vi "Read Cal Data.vi"(5 "NewOffsets(V)":dbl[](array[numeric]), 11 "error in (no error)":errorcluster, 12 "Enum":enum16{"Init", "Read", "Write"}(ring)) -> (4 "AllowZero":bool[](array[boolean]), 6 "Slope":dbl[](array[numeric]), 8 "Offset":dbl[](array[numeric]), 10 "Channel Names":string[](array[string]), 15 "error out":errorcluster)   [LabVIEW 2018]
uses:
  <vilib>/Utility/file.llb/Read Delimited Spreadsheet (string).vi
  <vilib>/Utility/file.llb/Write Delimited Spreadsheet (string).vi
panel:
  out "all rows":string[][](array[string])
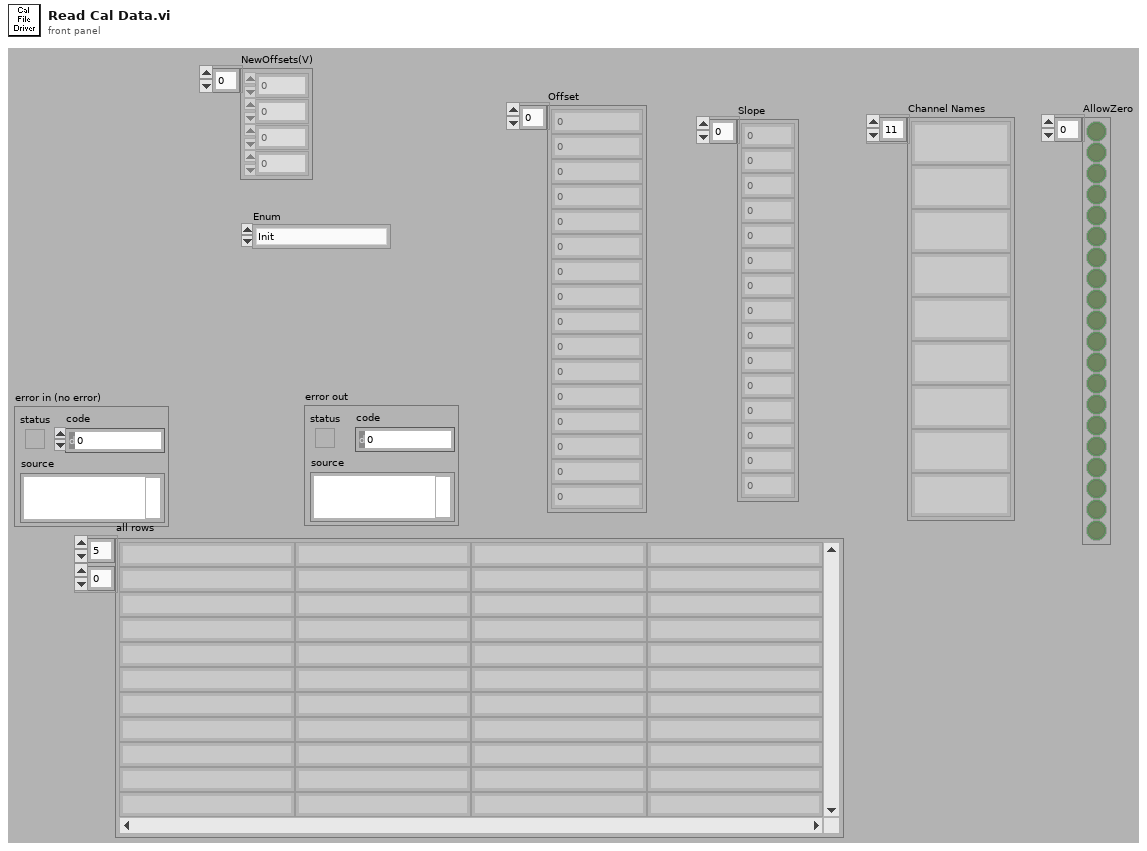
[diagram p1: front panel]
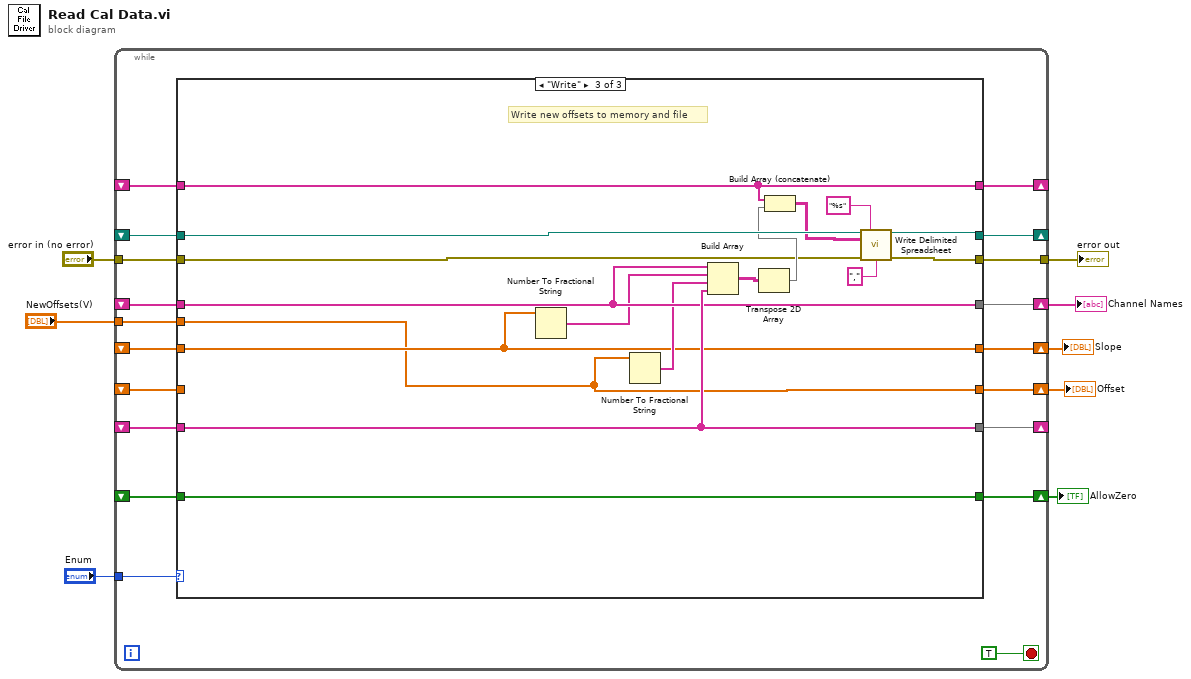
[diagram p0: block diagram]
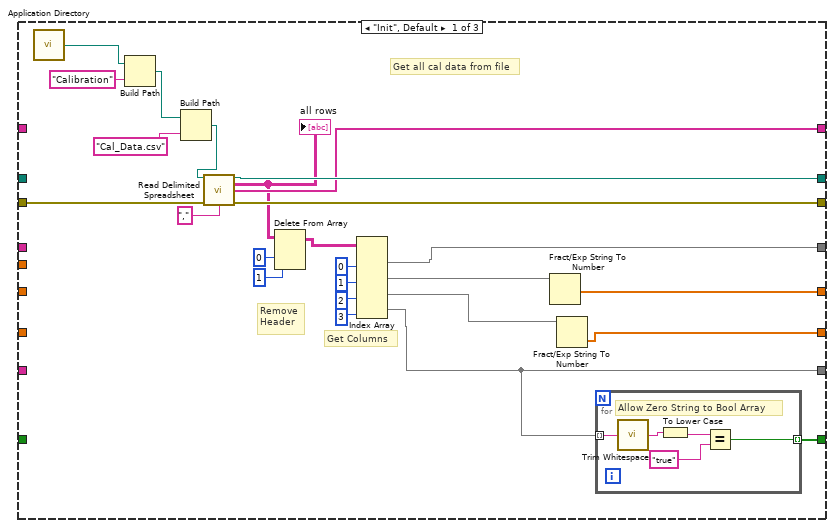
[diagram p2: hidden frame]
diagram:
  n1 = while {
    tunnel: "Enum" -> [w26]
    shift-right: [w25] -> w5
    shift-left: _ -> [w22]
    shift-right: [w24] -> w4
    shift-left: _ -> [w21]
    shift-right: [w23] -> w3
    shift-left: _ -> [w20]
    tunnel: "error in (no error)" -> [w18]
    tunnel: [w17] -> w8
    shift-right: [w16] -> _
    shift-left: _ -> [w19]
    shift-right: [w15] -> _
    shift-left: _ -> [w14]
    shift-right: [w13] -> _
    shift-left: _ -> [w12]
    tunnel: "NewOffsets(V)" -> [w11]
    shift-right: [w10] -> w1
    shift-left: _ -> [w9]
    stop <- TRUE stop-if-true
    n2 = case shown="\"Write\"" w26 {
      tunnel: [w44 w65 w66] -> w25
      tunnel: [w43 w64 w67] -> w24
      tunnel: [w32 w63 w71] -> w23
      tunnel: w22 -> [_ w65 _]
      tunnel: w21 -> [_ w64 w67]
      tunnel: w20 -> [_ w63 w71]
      tunnel: w19 -> [_ w62 w81]
      tunnel: w18 -> [w52 w58 w73]
      tunnel: [w51 w58 w77] -> w17
      tunnel: [w50 w62 w80] -> w16
      tunnel: [w29 w61 w76] -> w15
      tunnel: w14 -> [_ w61 w76]
      tunnel: [w37 w60 w72] -> w13
      tunnel: w12 -> [_ w60 w72]
      tunnel: w11 -> [_ _ w66]
      tunnel: [w28 w59 w68] -> w10
      tunnel: w9 -> [_ w59 w68]
      frame "Init", Default {
        # "Get Columns"
        # "Remove\nHeader"
        # "Get all cal data from file"
        n3 = call <vilib>:"Application Directory.vi"() -> ("Application Directory"=w40:path)
        n4 = Build Path(base path=w40, name or relative path="Calibration") -> (appended path=w38:path)
        n5 = Build Path(base path=w38, name or relative path="Cal_Data.csv") -> (appended path=w41:path)
        n6 = call-poly <vilib>:"Read Delimited Spreadsheet.vi"("file path (dialog if empty)"=w41, "error in (no error)"=w52, "delimiter (\\t)"="," ("delimiter (\\t)")) -> ("new file path (Not A Path if cancelled)"=w50:path, "all rows"=w34:string[][], "first row"=w37:string[], "error out"=w51:errorcluster)  [unwired: 7 in, 2 out]
        "all rows" <- w34
        n7 = Delete From Array(array=w34, length=1, index (row)=0) -> (array with subset deleted=w33:string[][])  [unwired: 1 in, 1 out]
        n8 = Index Array(array=w33, index (col) #1=0 ("disabled index (col)"), index (col) #2=1 ("index (col)"), index (col) #3=2 ("disabled index (col)"), index (col) #4=3 ("index (col)")) -> (element #1=w32:string[], element #2=w31:string[], element #3=w30:string[], element #4=w29:string[])  [unwired: 4 in]
        n9 = Fract/Exp String To Number(string=w31) -> (number=w43:dbl[])  [unwired: 3 in, 1 out]
        n10 = Fract/Exp String To Number(string=w30) -> (number=w44:dbl[])  [unwired: 3 in, 1 out]
        n11 = for {
          tunnel: w29 -> [w57] mode=indexing
          tunnel: [w53] -> w28 mode=indexing
          # "Allow Zero String to Bool Array"
          n12 = call <vilib>:"Trim Whitespace.vi"("string"=w57) -> ("trimmed string"=w56:string)  [unwired: 1 in]
          n13 = To Lower Case(string=w56) -> (all lower case string=w55:string)
          n14 = Equal?(x=w55, y="true") -> (x = y?=w53:bool)
        }
      }
      frame "Read" {
        # "Read the current values"
      }
      frame "Write" {
        # "Write new offsets to memory and file"
        n15 = Number To Fractional String(number=w67) -> (F-format string=w70:string[])  [unwired: 3 in]
        n16 = Number To Fractional String(number=w66) -> (F-format string=w69:string[])  [unwired: 3 in]
        n17 = Build Array(w71, w70, w69, w76) -> (w82:string[][])
        n18 = Transpose 2D Array(2D array=w82) -> (transposed array=w74:string[][])
        n19 = Build Array (concatenate)(w72, w74) -> (w75:string[][])
        n20 = call-poly <vilib>:"Write Delimited Spreadsheet.vi"("file path (dialog if empty)"=w81, "format (%s)"="%s" ("format (%.3f)"), "2D data"=w75, "error in (no error)"=w73, "delimiter (\\t)"="," ("delimiter (\\t)")) -> ("new file path (Not A Path if cancelled)"=w80:path, "error out"=w77:errorcluster)  [unwired: 9 in]
      }
    }
  }
  "error out" <- w8
  "Channel Names" <- w3
  "Offset" <- w5
  "Slope" <- w4
  "AllowZero" <- w1
